vi "BuildApplicationCmdLine.vi"() -> ()   [LabVIEW 2018]
uses:
  <vilib>/Wiresmith Technology/LabVIEW CLI/CLI Class/CLI.lvclass
panel:
  out "error out":errorcluster
  out "Generated files":path[](array[path])
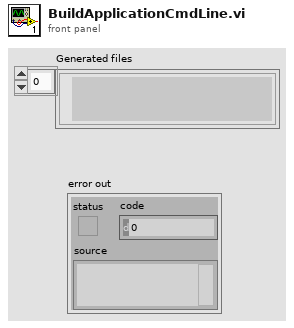
[diagram p1: front panel]
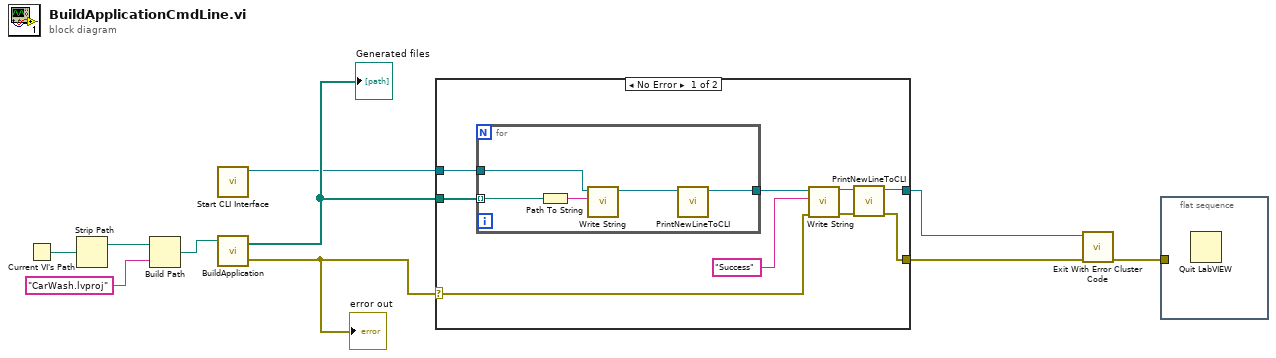
[diagram p0: block diagram]
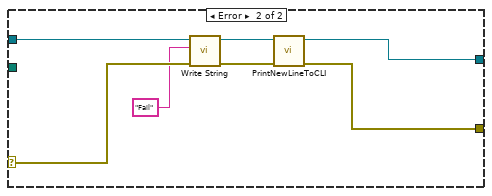
[diagram p2: hidden frame]
diagram:
  n1 = Current VI's Path() -> (path=w5:path)
  n2 = Strip Path(path=w5) -> (stripped path=w4:path)  [unwired: 1 out]
  n3 = Build Path(base path=w4, name or relative path="CarWash.lvproj") -> (appended path=w2:path)
  n4 = call <vilib>:"Start CLI Interface.vi"() -> ("CLI out"=w9:refnum<class "CLI.lvclass">)  [unwired: 9 in, 2 out]
  n5 = call "BuildApplication.vi"("Path to project"=w2) -> ("error out"=w7:errorcluster, "Generated files"=w10:path[])  [unwired: 2 in]
  "Generated files" <- w10
  "error out" <- w7
  n6 = case shown="No Error" w7 {
    selector: w7 -> [w16 w30]
    tunnel: w10 -> [w19 _]
    tunnel: w9 -> [w18 w31]
    tunnel: [w11 w26] -> w8
    tunnel: [w12 w25] -> w6
    frame No Error {
      n7 = for {
        tunnel: w19 -> [w23] mode=indexing
        tunnel: w18 -> [w24]
        tunnel: [w20] -> w17
        n8 = Path To String(path=w23) -> (string=w22:string)
        n9 = call <vilib>:"Write String.vi"("Text to Write"=w22, "CLI in"=w24) -> ("CLI out"=w21:refnum<class "CLI.lvclass">)  [unwired: 8 in, 1 out]
        n10 = call "PrintNewLineToCLI.vi"("CLI in"=w21) -> ("CLI out"=w20:refnum<class "CLI.lvclass">)  [unwired: 9 in, 1 out]
      }
      n11 = call <vilib>:"Write String.vi"("error in (no error)"=w16, "Text to Write"="Success", "CLI in"=w17) -> ("error out"=w13:errorcluster, "CLI out"=w14:refnum<class "CLI.lvclass">)  [unwired: 7 in]
      n12 = call "PrintNewLineToCLI.vi"("error in (no error)"=w13, "CLI in"=w14) -> ("error out"=w12:errorcluster, "CLI out"=w11:refnum<class "CLI.lvclass">)  [unwired: 8 in]
    }
    frame Error {
      n13 = call <vilib>:"Write String.vi"("error in (no error)"=w30, "Text to Write"="Fail", "CLI in"=w31) -> ("error out"=w27:errorcluster, "CLI out"=w28:refnum<class "CLI.lvclass">)  [unwired: 7 in]
      n14 = call "PrintNewLineToCLI.vi"("error in (no error)"=w27, "CLI in"=w28) -> ("error out"=w25:errorcluster, "CLI out"=w26:refnum<class "CLI.lvclass">)  [unwired: 8 in]
    }
  }
  n15 = call <vilib>:"Exit With Error Cluster Code.vi"("error in (no error)"=w6, "CLI in"=w8) -> ("error out"=w1:errorcluster)  [unwired: 9 in]
  n16 = flat-sequence {
    tunnel: w1 -> [_]
    frame #0 {
      n17 = Quit LabVIEW() -> ()  [unwired: 1 in]
    }
  }
